vi "Initial XY (SubVI).vi"(1 "Mode initial 2D":enum32{"2D", "X"}(radio), 2 "error in":errorcluster, 3 "VISA Refnum in":refnum<visa-resource-name>) -> (0 "error out":errorcluster)   [LabVIEW 2018]
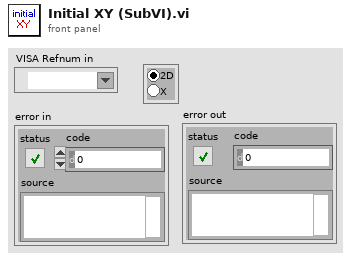
[diagram p1: front panel]
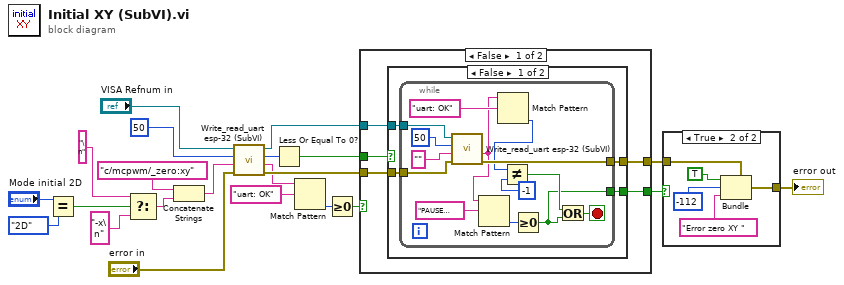
[diagram p0: block diagram]
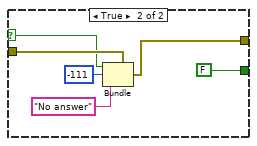
[diagram p2: hidden frame]
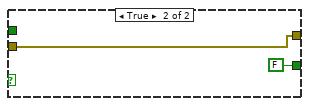
[diagram p3: hidden frame]
diagram:
  n1 = Equal?(x="Mode initial 2D", y=enum32{"2D", "X"}."2D" ("Mode initial 2D")) -> (x = y?=w4:bool)
  n2 = Select(t="\n", s=w4, f="-x\n") -> (s? t:f=w1:string)
  n3 = Concatenate Strings("c/mcpwm/_zero:xy" ("write buffer"), w1) -> (w8:string)
  n4 = call "Write_read_uart esp-32 (SubVI).vi"("error in (no error)"="error in", "write buffer"=w8, "milliseconds to wait"=u32 50, "VISA Refnum in"="VISA Refnum in") -> ("error out 4"=w22:errorcluster, "read buffer"=w11:string, "read bite"=w13:u32, "VISA resource name out"=w21:refnum<visa-resource-name>)
  n5 = Less Or Equal To 0?(x=w13) -> (x <= 0?=w20:bool)
  n6 = Match Pattern(string=w11, regular expression="uart: OK") -> (offset past match=w10:i32)  [unwired: 1 in, 3 out]
  n7 = Greater Or Equal To 0?(x=w10) -> (x >= 0?=w9:bool)
  n8 = case shown="False" w9 {
    tunnel: w22 -> [w27 w53]
    tunnel: w21 -> [w26 _]
    tunnel: w20 -> [w25 _]
    tunnel: [w24 w53] -> w17
    tunnel: [w23 FALSE] -> w16
    frame False {
      n9 = case shown="False" w25 {
        selector: w25 -> [_ w49]
        tunnel: w27 -> [w31 w50]
        tunnel: w26 -> [w30 _]
        tunnel: [w29 w46] -> w24
        tunnel: [w28 FALSE] -> w23
        frame False {
          n10 = while {
            tunnel: w31 -> [w43]
            tunnel: w30 -> [w42]
            tunnel: [w38] -> w29
            tunnel: [w32] -> w28
            stop <- w39 stop-if-true
            n11 = call "Write_read_uart esp-32 (SubVI).vi"("error in (no error)"=w43, "write buffer"="", "milliseconds to wait"=u32 50, "VISA Refnum in"=w42) -> ("error out 4"=w38:errorcluster, "read buffer"=w35:string)  [unwired: 2 out]
            n12 = Match Pattern(string=w35, regular expression="PAUSE rotate") -> (offset past match=w33:i32)  [unwired: 1 in, 3 out]
            n13 = Match Pattern(string=w35, regular expression="uart: OK") -> (offset past match=w37:i32)  [unwired: 1 in, 3 out]
            n14 = Not Equal?(x=w37, y=-1 ("offset past match")) -> (x != y?=w36:bool)
            n15 = Greater Or Equal To 0?(x=w33) -> (x >= 0?=w32:bool)
            n16 = Or(x=w36, y=w32) -> (x .or. y?=w39:bool)
          }
        }
        frame True {
          n17 = Bundle(cluster=w50, "status"=w49, "code"=-111, "source"="No answer") -> (w46:errorcluster)
        }
      }
    }
    frame True {
    }
  }
  n18 = case shown="True" w16 {
    tunnel: w17 -> [w54 w58]
    tunnel: [w54 w55] -> w15
    frame False {
    }
    frame True {
      n19 = Bundle(cluster=w58, "status"=TRUE, "code"=-112, "source"="Error zero XY ") -> (w55:errorcluster)
    }
  }
  "error out" <- w15
